vi "Seconds Format String.vi"(10 "Unit (ms)":T1=enum."millisecond") -> (2 "format string":string)   [LabVIEW 2013]
uses:
  Seconds Units -- enum.ctl
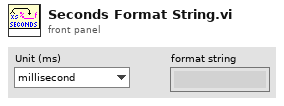
[diagram p1: front panel]
types:
  T1 = typedef "Seconds Units -- enum.ctl" = enum16{"second", "millisecond", "microsecond", "nanosecond"}
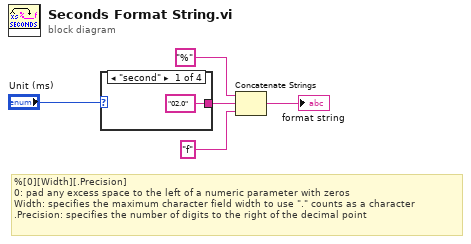
[diagram p0: block diagram]
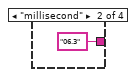
[diagram p2: hidden frame]
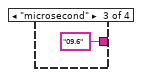
[diagram p3: hidden frame]
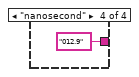
[diagram p4: hidden frame]
diagram:
  # "%[0][Width][.Precision]\n0: pad any excess space to the left of a numeric parameter with zeros\nWidth: specifies the maximum character field width to use \".\" counts as a character\n.Precision: specifies the number of digits to the right of the decimal point"
  n1 = case shown="\"second\"" "Unit (ms)" {
    tunnel: ["02.0" "06.3" "09.6" "012.9"] -> w3
    frame "second" {
    }
    frame "millisecond" {
    }
    frame "microsecond" {
    }
    frame "nanosecond" {
    }
  }
  n2 = Concatenate Strings("%", w3, "f") -> (→"format string":string)
